vi "Queue Driver.vi"(0 "State and data":T1[](array[typedef]), 2 "Name":string, 11 "Error in":errorcluster, 13 "Queue Operations":T2) -> (4 "Dequeued output":T1, 15 "Error out":errorcluster)   [LabVIEW 2020, in "PSRR Monitor.lvlib"]
doc: "This subvi is used as a queue driver for a producer consumer based state machine"
uses:
  PSRR Monitor.lvlib
  Typedefs/Queue operations.ctl
  Typedefs/Variant cluster.ctl
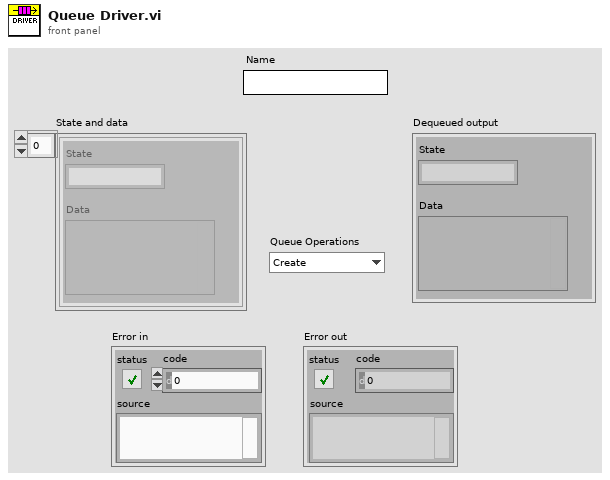
[diagram p1: front panel]
types:
  T1 = typedef "PSRR Monitor.lvlib/Variant cluster.ctl" = cluster{"State":string, "Data":variant}
  T2 = typedef "PSRR Monitor.lvlib/Queue operations.ctl" = enum16{"Create", "Enqueue", "Enstack", "Dequeue", "Flush", "Release "}
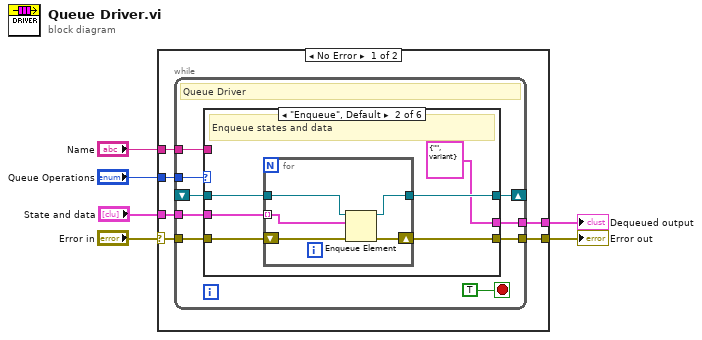
[diagram p0: block diagram]
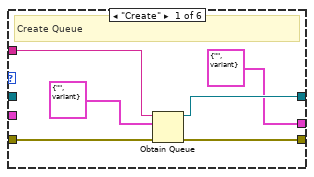
[diagram p2: hidden frame]
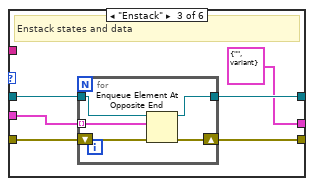
[diagram p3: hidden frame]
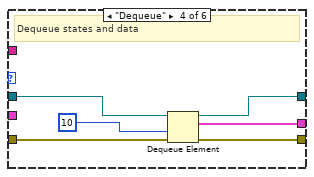
[diagram p4: hidden frame]
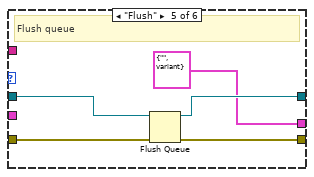
[diagram p5: hidden frame]
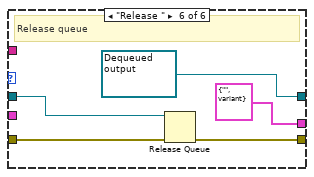
[diagram p6: hidden frame]
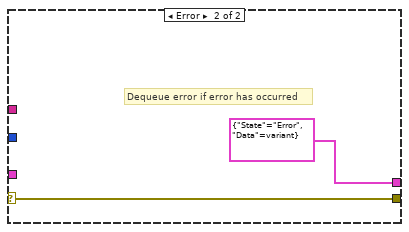
[diagram p7: hidden frame]
diagram:
  n1 = case shown="No Error" "Error in" {
    selector: "Error in" -> [w11 w67]
    tunnel: "Queue Operations" -> [w12 _]
    tunnel: [w10 w67] -> w4
    tunnel: "State and data" -> [w9 _]
    tunnel: "Name" -> [w8 _]
    tunnel: [w7 T1 {"State"="Error", "Data"=variant} ("Dequeued output")] -> w1
    frame No Error {
      n2 = while {
        tunnel: w12 -> [w20]
        tunnel: w11 -> [w19]
        tunnel: [w18] -> w10
        tunnel: w9 -> [w17]
        shift-right: [w15] -> _
        shift-left: _ -> [w16]
        tunnel: w8 -> [w14]
        tunnel: [w13] -> w7
        stop <- TRUE stop-if-true
        # "Queue Driver"
        n3 = case shown="\"Enqueue\", Default" w20 {
          tunnel: w19 -> [w27 w33 w44 w55 w60 w65]
          tunnel: [w26 w32 w43 w54 w59 w64] -> w18
          tunnel: w17 -> [_ w31 w42 _ _ _]
          tunnel: w16 -> [_ w30 w41 w52 w58 w63]
          tunnel: [w24 w29 w40 w53 w57 refnum<queue> refnum ("queue out")] -> w15
          tunnel: w14 -> [w25 _ _ _ _ _]
          tunnel: [T1 {"State"="", "Data"=variant} ("Dequeued output") T1 {"State"="", "Data"=variant} ("Dequeued output") T1 {"State"="", "Data"=variant} ("Dequeued output") w51 T1 {"State"="", "Data"=variant} ("Dequeued output") T1 {"State"="", "Data"=variant} ("Dequeued output")] -> w13
          frame "Create" {
            # "Create Queue"
            n4 = Obtain Queue(name (unnamed)=w25, element data type=T1 {"State"="", "Data"=variant} ("Dequeued output"), error in (no error)=w27) -> (queue out=w24:refnum<queue>, error out=w26:errorcluster)  [unwired: 2 in, 1 out]
          }
          frame "Enqueue", Default {
            # "Enqueue states and data"
            n5 = for {
              shift-right: [w37] -> w32
              shift-left: w33 -> [w38]
              tunnel: w31 -> [w34] mode=indexing
              tunnel: [w36] -> w29
              tunnel: w30 -> [w35]
              n6 = Enqueue Element(queue=w35, element=w34, error in (no error)=w38) -> (queue out=w36:refnum<queue>, error out=w37:errorcluster)  [unwired: 1 in, 1 out]
            }
          }
          frame "Enstack" {
            # "Enstack states and data"
            n7 = for {
              shift-right: [w48] -> w43
              shift-left: w44 -> [w49]
              tunnel: w42 -> [w47] mode=indexing
              tunnel: w41 -> [w46]
              tunnel: [w45] -> w40
              n8 = Enqueue Element At Opposite End(queue=w46, element=w47, error in (no error)=w49) -> (queue out=w45:refnum<queue>, error out=w48:errorcluster)  [unwired: 1 in, 1 out]
            }
          }
          frame "Dequeue" {
            # "Dequeue states and data"
            n9 = Dequeue Element(queue=w52, timeout in ms (-1)=10, error in (no error)=w55) -> (queue out=w53:refnum<queue>, element=w51:T1, error out=w54:errorcluster)  [unwired: 1 out]
          }
          frame "Flush" {
            # "Flush queue"
            n10 = Flush Queue(queue=w58, error in (no error)=w60) -> (queue out=w57:refnum<queue>, error out=w59:errorcluster)  [unwired: 1 out]
          }
          frame "Release " {
            # "Release queue"
            n11 = Release Queue(queue=w63, error in (no error)=w65) -> (error out=w64:errorcluster)  [unwired: 1 in, 2 out]
          }
        }
      }
    }
    frame Error {
      # "Dequeue error if error has occurred"
    }
  }
  "Error out" <- w4
  "Dequeued output" <- w1
